vi "scale and decimate.vi"(9 "scale":T1, 10 "Waveform in":waveform(dbl), 11 "decimating factor":i32) -> (3 "Waveform out":waveform(dbl))   [LabVIEW 2014, in "PLS Acquisition.lvlib"]
uses:
  PLS Acquisition.lvlib
  Settings/conversion.ctl
  <vilib>/Analysis/2dsp.llb/Decimate (single shot, DBL).vi
  <vilib>/Analysis/NI_AALPro.lvlib
  Settings/PLS Settings.lvlib
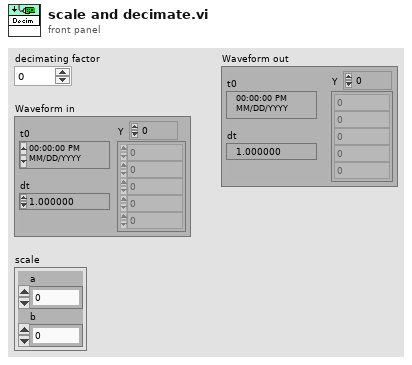
[diagram p1: front panel]
types:
  T1 = typedef "PLS Settings.lvlib/conversion.ctl" = cluster{"a":dbl, "b":dbl}
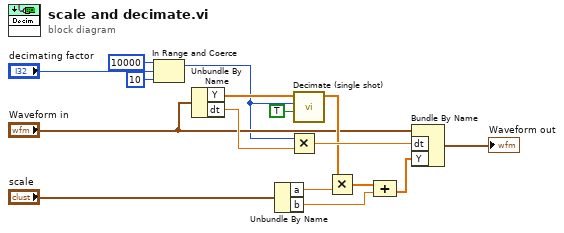
[diagram p0: block diagram]
diagram:
  n1 = In Range and Coerce(upper limit=10000, x="decimating factor", lower limit=10) -> (coerced(x)=w1:i32)  [unwired: 1 out]
  n2 = Unbundle By Name("Waveform in") -> ("Y"=w14:dbl[], "dt"=w15:dbl)
  n3 = Unbundle By Name("scale") -> ("a"=w6:dbl, "b"=w8:dbl)
  n4 = Multiply(x=w1, y=w15) -> (x*y=w16:dbl)
  n5 = call-poly <vilib>:"Decimate (single shot).vi"("averaging"=TRUE, "decimating factor"=w1, "X"=w14) -> ("Decimated Array"=w12:dbl[])  [unwired: 7 in, 1 out]
  n6 = Multiply(x=w12, y=w6) -> (x*y=w7:dbl[])
  n7 = Compound Arithmetic op=ADD(w7, w8) -> (w13:dbl[])
  n8 = Bundle By Name(cluster="Waveform in", "dt"=w16, "Y"=w13) -> (→"Waveform out":waveform(dbl))
